vi "Colors_of_z-Axis.vi"(0 "Array":dbl[][](array[numeric])=[[1.0, 2.0, 3.0, 4.0, 5.0], [6.0, 7.0, 8.0, 9.0, 10.0], [11.0, 12.0, 13.0, 14.0, 15.0], [16.0, 17.0, 18.0, 19.0, 20.0]], 1 "scaling":u16(ring)=1 items=["logarithmic", "linear"], 2 "Y Scale.Range:Maximum":u32=4, 3 "Y Scale.Range:Minimum":u32=1, 4 "X Scale.Range:Maximum":u32=3, 5 "X Scale.Range:Minimum":u32, 7 "complete array":bool) -> (14 "Colors":cluster{dbl, u32}[](array[cluster])=[{20.0, 16448250}, {16.826999999999998, 16711680}, {13.673, 16776960}, {10.5, 6618880}, {7.327, 16860}, {4.173, 8388863}, {1.0, 0}], 15 "Maximum":dbl=20.0, 16 "Minimum":dbl=1.0)   [LabVIEW 2013]
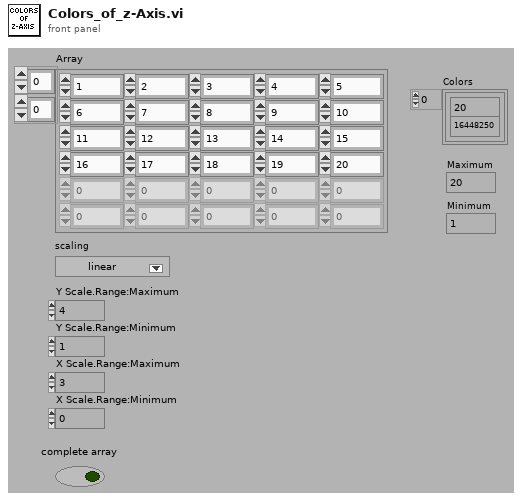
[diagram p1: front panel]
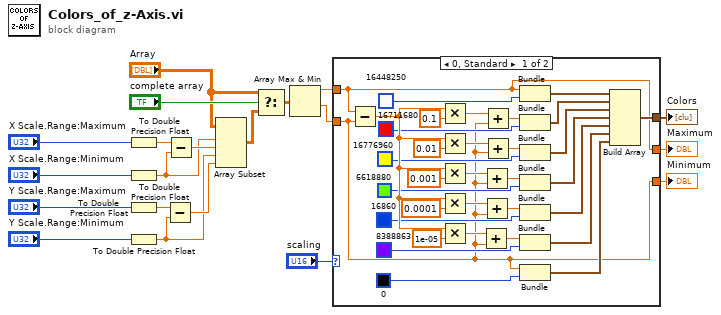
[diagram p0: block diagram]
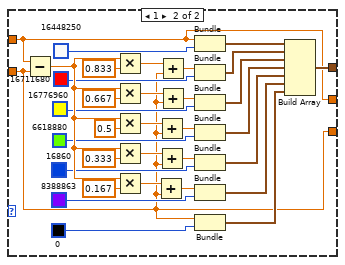
[diagram p2: hidden frame]
diagram:
  n1 = To Double Precision Float(number="X Scale.Range:Maximum") -> (double precision float=w1:dbl)
  n2 = To Double Precision Float(number="X Scale.Range:Minimum") -> (double precision float=w3:dbl)
  n3 = To Double Precision Float(number="Y Scale.Range:Maximum") -> (double precision float=w5:dbl)
  n4 = To Double Precision Float(number="Y Scale.Range:Minimum") -> (double precision float=w7:dbl)
  n5 = Subtract(x=w5, y=w7) -> (x-y=w13:dbl)
  n6 = Subtract(x=w1, y=w3) -> (x-y=w14:dbl)
  n7 = Array Subset(array="Array", index (row)=w3, length (row)=w14, index (col)=w7, length (col)=w13) -> (w10:dbl[][])
  n8 = Select(t="Array", s="complete array", f=w10) -> (s? t:f=w9:dbl[][])
  n9 = Array Max & Min(array=w9) -> (max value=w19:dbl, min value=w18:dbl)  [unwired: 2 out]
  n10 = case shown="0, Standard" "scaling" {
    tunnel: [w21 w54] -> w15
    tunnel: [w22 w55] -> w16
    tunnel: [w23 w56] -> w17
    tunnel: w19 -> [w22 w55]
    tunnel: w18 -> [w21 w54]
    frame 0, Default {
      n11 = Subtract(x=w22, y=w21) -> (x-y=w43:dbl)
      n12 = Multiply(x=w43, y=0.1) -> (x*y=w45:dbl)
      n13 = Multiply(x=w43, y=0.01) -> (x*y=w47:dbl)
      n14 = Multiply(x=w43, y=0.001) -> (x*y=w49:dbl)
      n15 = Multiply(x=w43, y=0.0001) -> (x*y=w51:dbl)
      n16 = Multiply(x=w43, y=1e-05) -> (x*y=w53:dbl)
      n17 = Add(x=w53, y=w21) -> (x+y=w44:dbl)
      n18 = Add(x=w49, y=w21) -> (x+y=w50:dbl)
      n19 = Add(x=w51, y=w21) -> (x+y=w52:dbl)
      n20 = Add(x=w45, y=w21) -> (x+y=w46:dbl)
      n21 = Add(x=w47, y=w21) -> (x+y=w48:dbl)
      n22 = Bundle(w22, u32 16448250) -> (w36:cluster{dbl, u32})  [unwired: 1 in]
      n23 = Bundle(w46, u32 16711680) -> (w37:cluster{dbl, u32})  [unwired: 1 in]
      n24 = Bundle(w48, u32 16776960) -> (w38:cluster{dbl, u32})  [unwired: 1 in]
      n25 = Bundle(w50, u32 6618880) -> (w39:cluster{dbl, u32})  [unwired: 1 in]
      n26 = Bundle(w52, u32 16860) -> (w40:cluster{dbl, u32})  [unwired: 1 in]
      n27 = Bundle(w44, u32 8388863) -> (w41:cluster{dbl, u32})  [unwired: 1 in]
      n28 = Bundle(w21, u32 0) -> (w42:cluster{dbl, u32})  [unwired: 1 in]
      n29 = Build Array(w36, w37, w38, w39, w40, w41, w42) -> (w23:cluster{dbl, u32}[])
    }
    frame 1 {
      n30 = Subtract(x=w55, y=w54) -> (x-y=w76:dbl)
      n31 = Multiply(x=w76, y=0.833) -> (x*y=w78:dbl)
      n32 = Multiply(x=w76, y=0.667) -> (x*y=w80:dbl)
      n33 = Multiply(x=w76, y=0.5) -> (x*y=w82:dbl)
      n34 = Multiply(x=w76, y=0.333) -> (x*y=w84:dbl)
      n35 = Multiply(x=w76, y=0.167) -> (x*y=w86:dbl)
      n36 = Add(x=w86, y=w54) -> (x+y=w77:dbl)
      n37 = Add(x=w82, y=w54) -> (x+y=w83:dbl)
      n38 = Add(x=w84, y=w54) -> (x+y=w85:dbl)
      n39 = Add(x=w78, y=w54) -> (x+y=w79:dbl)
      n40 = Add(x=w80, y=w54) -> (x+y=w81:dbl)
      n41 = Bundle(w55, u32 16448250) -> (w69:cluster{dbl, u32})  [unwired: 1 in]
      n42 = Bundle(w79, u32 16711680) -> (w70:cluster{dbl, u32})  [unwired: 1 in]
      n43 = Bundle(w81, u32 16776960) -> (w71:cluster{dbl, u32})  [unwired: 1 in]
      n44 = Bundle(w83, u32 6618880) -> (w72:cluster{dbl, u32})  [unwired: 1 in]
      n45 = Bundle(w85, u32 16860) -> (w73:cluster{dbl, u32})  [unwired: 1 in]
      n46 = Bundle(w77, u32 8388863) -> (w74:cluster{dbl, u32})  [unwired: 1 in]
      n47 = Bundle(w54, u32 0) -> (w75:cluster{dbl, u32})  [unwired: 1 in]
      n48 = Build Array(w69, w70, w71, w72, w73, w74, w75) -> (w56:cluster{dbl, u32}[])
    }
  }
  "Colors" <- w17
  "Minimum" <- w15
  "Maximum" <- w16
